vi "LV Basics I.vi"() -> ()   [LabVIEW 2015]
doc: "Use this template to simulate the generation and display of data.\nNote: LabVIEW enables automatic error handling by default for VIs you create from this template."
uses:
  Instance           1 27Saved   GenerateDisplay.vit .vi
panel:
  in  "Amplitude":dbl(knob) scale=0.0..5.0
  in  "Numeric":dbl
  out "Waveform Graph":dynamicdata(graph)
  in  "stop":bool
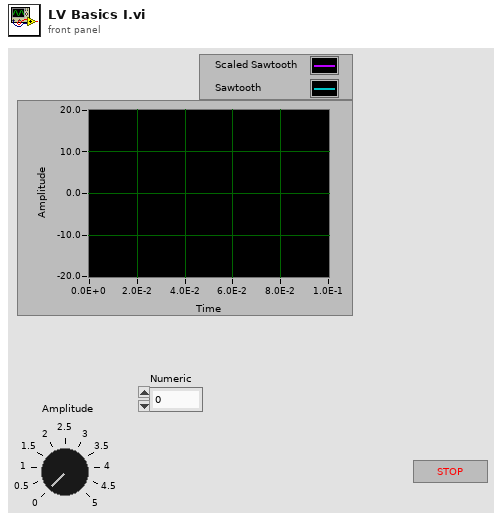
[diagram p1: front panel]
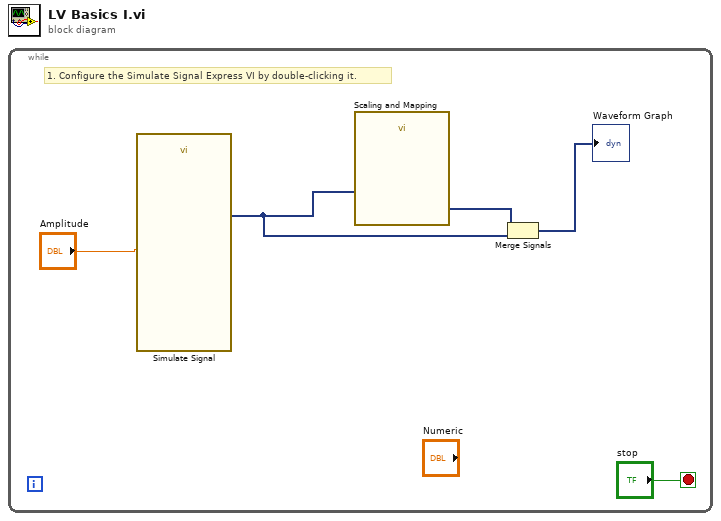
[diagram p0: block diagram]
diagram:
  n1 = while {
    stop <- "stop" stop-if-true
    # "1. Configure the Simulate Signal Express VI by double-clicking it."
    n2 = call "Simulate Signal"("Amplitude"="Amplitude") -> ("Sawtooth"=w2:dynamicdata)  [unwired: 13 in, 1 out]
    n3 = call "Scaling and Mapping"("Signals"=w2) -> ("Scaled Signals"=w3:dynamicdata)  [unwired: 9 in, 1 out]
    n4 = Merge Signals(w3, w2) -> (→"Waveform Graph":dynamicdata)
  }
